vi "rxTrchDecoder.vi"(8 "error in":errorcluster, 10 "inputData":dbl[](array[numeric]), 11 "Path In":path) -> (0 "error out":errorcluster, 2 "out_data":dbl[](array[numeric]), 3 "Path Out":path)   [LabVIEW 2015]
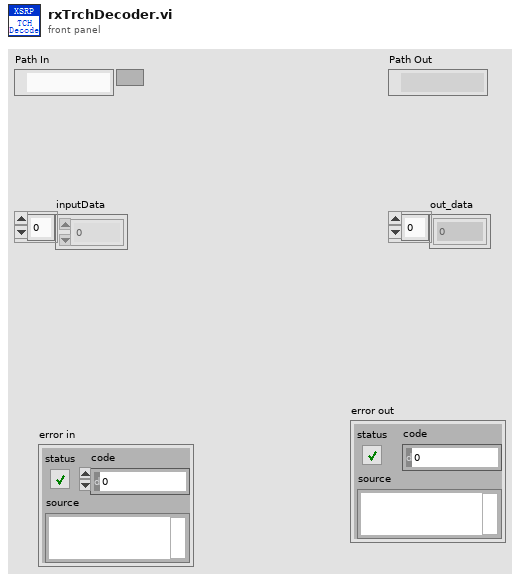
[diagram p1: front panel]
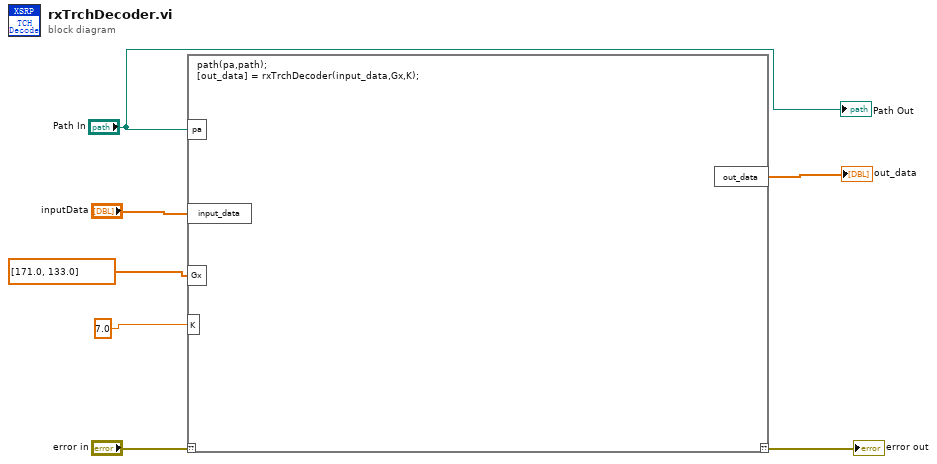
[diagram p0: block diagram]
diagram:
  n1 = script code="path(pa,path);\n[out_data] = rxTrchDecoder(input_data,Gx,K);"("??"="error in", "pa"="Path In", "input_data"="inputData", "Gx"=dbl[] [171.0, 133.0], "K"=7.0) -> ("??"=→"error out":errorcluster, "out_data"=→"out_data":dbl[])
  "Path Out" <- "Path In"
